vi "Stop Test.vi"(8 "error in (no error)":errorcluster, 10 "Stop Test":bool, 11 "Test Application Controller in":refnum<class "Test Application Controller.lvclass">) -> (0 "error out":errorcluster, 3 "Test Application Controller out":refnum<class "Test Application Controller.lvclass">)   [LabVIEW 2017, in "Test Application Controller.lvlib" / "Test Application Controller.lvclass"]
uses:
  Test Application Controller.lvclass
  Test Application Controller.lvclass/Test Application Controller.ctl
  <vilib>/ActorFramework/Message Enqueuer/Message Enqueuer.lvclass/Message Enqueuer.ctl
  <vilib>/ActorFramework/Message Enqueuer/Enqueue.vi
  <vilib>/ActorFramework/Stop Msg/Stop Msg.lvclass
  C:/Program Files (x86)/National Instruments/LabVIEW 2017/vi.lib/ActorFramework/Message/Message.lvclass
  <vilib>/ActorFramework/Message Priority Queue/Priority Enqueue.vi
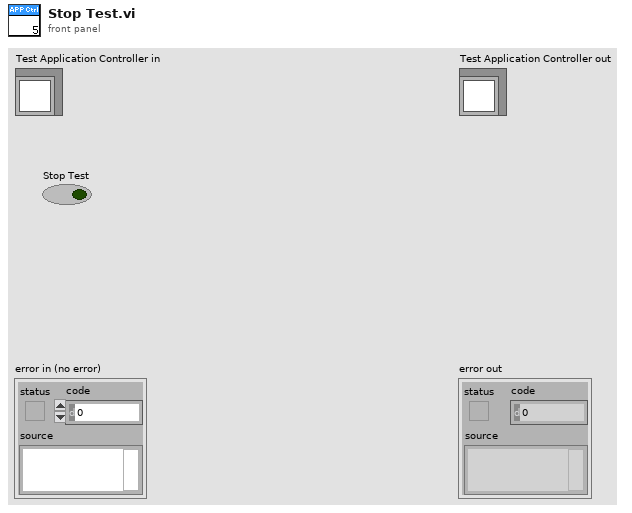
[diagram p1: front panel]
types:
  T1 = cluster{"Stop":refnum<user-event>, "Tests to Execute":refnum<user-event>, "Stop Test":refnum<user-event>, "Generate Report":refnum<user-event>, "Status String":refnum<user-event>}
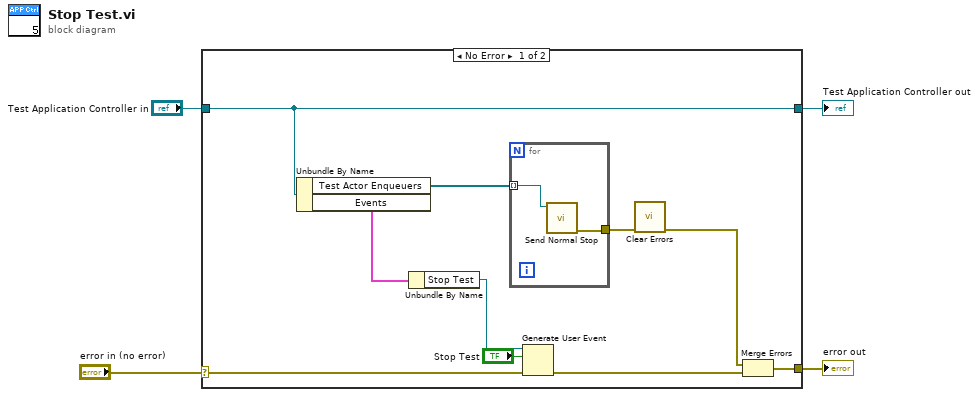
[diagram p0: block diagram]
diagram:
  n1 = case shown="No Error" "error in (no error)" {
    selector: "error in (no error)" -> [w13 w18]
    tunnel: [w6 w18] -> w3
    tunnel: [w14 w17] -> w1
    tunnel: "Test Application Controller in" -> [w14 w17]
    frame No Error {
      n2 = Unbundle By Name(w14) -> ("Test Actor Enqueuers"=w9:refnum<class "Message Enqueuer.lvclass">[], "Events"=w12:T1)
      n3 = Unbundle By Name(w12) -> ("Stop Test"=w11:refnum<user-event>)
      n4 = for {
        tunnel: w9 -> [w16] mode=indexing
        tunnel: [w15] -> w8
        n5 = call <vilib>:"Send Normal Stop.vi"("Message Enqueuer"=w16) -> ("error out"=w15:errorcluster)  [unwired: 10 in]
      }
      n6 = Generate User Event(user event=w11, event data cluster="Stop Test", error in=w13) -> (error out=w5:errorcluster)  [unwired: 1 in, 1 out]
      n7 = call <vilib>:"Clear Errors.vi"("error in (no error)"=w8) -> ("error out"=w7:errorcluster)  [unwired: 5 in, 1 out]
      n8 = Merge Errors(w7, w5) -> (w6:errorcluster)
    }
    frame Error {
    }
  }
  "error out" <- w3
  "Test Application Controller out" <- w1
